vi "Check key pressed.vi"(1 "Key pressed":T1) -> (0 "Enter was pressed?":bool)   [LabVIEW 2023]
uses:
  <vilib>/event_ctls.llb/eventvkey.ctl
panel:
  in  "Enter/return array":T1[](array[typedef])=[enum."Enter", enum."Return"]
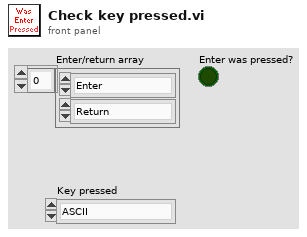
[diagram p1: front panel]
types:
  T1 = typedef "eventvkey.ctl" = enum16{"ASCII", "Enter", "Return", "Shift", "Ctrl", "Alt", "Cmd", "Opt", "Caps", "NumLock", "Clear", "Break", "Up", "Down", "Left", "Right", "Insert", "Delete", "Home", "End", "PageUp", "PageDown", "Escape", "Help", "Pause", "ScrollLock", "F1", "F2", "F3", "F4", "F5", "F6", "F7", "F8", "F9", "F10", "F11", "F12", "F13", "F14", "F15", "F16", "F17", "F18", "F19", "F20", "F21", "F22", "F23", "F24", "Play", "VolumeUp", "VolumeDown", "Mute", "Two Byte Char"}
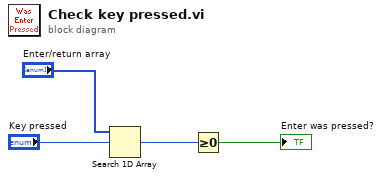
[diagram p0: block diagram]
diagram:
  n1 = Search 1D Array(1D array="Enter/return array", element="Key pressed") -> (index of element=w2:i32)  [unwired: 1 in]
  n2 = Greater Or Equal To 0?(x=w2) -> (x >= 0?=→"Enter was pressed?":bool)
